vi "ConfigChannels.vi"(8 "error in (no error)":errorcluster, 11 "NiDaqMx in":refnum<class "NiDaqMx.lvclass">) -> (0 "error out":errorcluster, 3 "NiDaqMx out":refnum<class "NiDaqMx.lvclass">)   [LabVIEW 2018, in "DigitizerPlugins.lvlib" / "NiDaqMx.lvclass"]
uses:
  NiDaqMx.lvclass
  X:/Projects/PMUCal/Modules/Digitizer/DigitizerPlugins/DigitizerBaseClass/DigitizerBase.lvclass
  DigitizerBaseClass/DigitizerBase.lvclass/DigitizerBase.ctl
  DigitizerBaseClass/Accessors/Read InstRef.vi
  DigitizerBaseClass/Accessors/Read Handle.vi
  DigitizerBaseClass/Accessors/Read Channels.vi
  DigitizerBaseClass/Accessors/Write InstRef.vi
  <vilib>/DAQmx/create/channels.llb/DAQmx Create Channel (AI-Voltage-Basic).vi
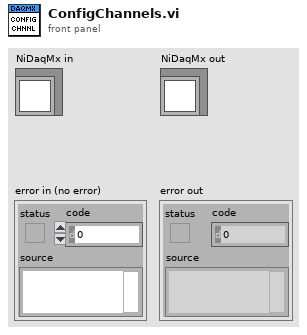
[diagram p1: front panel]
types:
  T1 = typedef "DigitizerPlugins.lvlib/DigitizerBase.lvclass/Channel.ctl" = cluster{"Name":string, "Enabled":bool, "InputImpedance":dbl, "Coupling":enum16{"AC", "DC", "Gnd"}, "Offset":dbl, "Range":dbl}
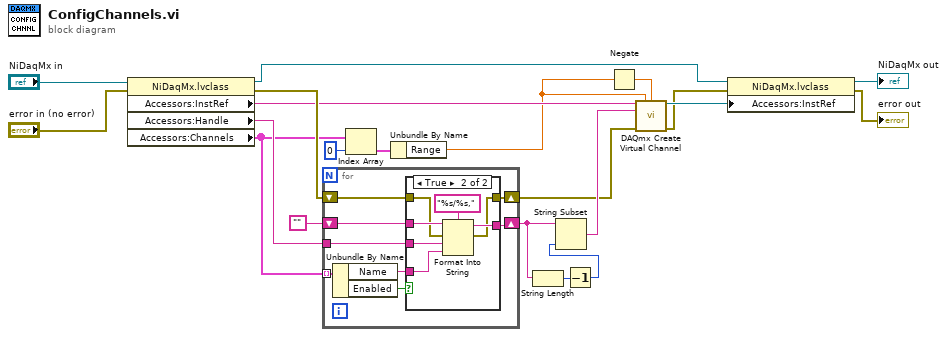
[diagram p0: block diagram]
diagram:
  n1 = property class="NiDaqMx.lvclass"(reference="NiDaqMx in", error in="error in (no error)") -> (reference out=w6:refnum<class "NiDaqMx.lvclass">, error out=w18:errorcluster, "Accessors:InstRef"=w14:string, "Accessors:Handle"=w20:string, "Accessors:Channels"=w12:T1[])
  n2 = for {
    tunnel: w12 -> [w27] mode=indexing
    tunnel: w20 -> [w28]
    shift-right: [w25] -> w17
    shift-left: "" -> [w29]
    shift-right: [w23] -> w7
    shift-left: w18 -> [w24]
    n3 = Unbundle By Name(w27) -> ("Name"=w26:string, "Enabled"=w22:bool)
    n4 = case shown="True" w22 {
      tunnel: w29 -> [w30 w38]
      tunnel: w28 -> [_ w36]
      tunnel: w26 -> [_ w35]
      tunnel: [w30 w34] -> w25
      tunnel: w24 -> [w31 w33]
      tunnel: [w31 w32] -> w23
      frame False {
      }
      frame True {
        n5 = Format Into String(format string="%s/%s,", initial string=w38, error in=w33, w36, w35) -> (resulting string=w34:string, error out=w32:errorcluster)
      }
    }
  }
  n6 = Index Array(array=w12, index=0) -> (element=w10:T1)
  n7 = Unbundle By Name(w10) -> ("Range"=w8:dbl)
  n8 = String Length(string=w17) -> (length=w16:i32)
  n9 = Decrement(x=w16) -> (x-1=w15:i32)
  n10 = String Subset(string=w17, length (rest)=w15) -> (substring=w13:string)  [unwired: 1 in]
  n11 = Negate(x=w8) -> (-x=w9:dbl)
  n12 = call-poly <vilib>:"DAQmx Create Virtual Channel.vi"("task in"=w14, "maximum value"=w8, "minimum value"=w9, "physical channels"=w13, "error in"=w7) -> ("task out"=w5:refnum<k21>, "error out"=w4:errorcluster)  [unwired: 9 in]
  n13 = property class="NiDaqMx.lvclass"(reference=w6, error in=w4, "Accessors:InstRef"=w5) -> (reference out=→"NiDaqMx out":refnum<class "NiDaqMx.lvclass">, error out=→"error out":errorcluster)
